vi "Find RetVal Wire_UNUSED.vi"(8 "Error In":errorcluster, 11 "Proto Method VI":refnum<vi>) -> (0 "Error Out":errorcluster, 2 "RetVal Wire":refnum<vi>, 3 "Proto Method VI Dup":refnum<vi>)   [LabVIEW 2013, in "Abstract Param Writer.lvclass"]
uses:
  Abstract Param Writer.lvclass
  <vilib>/Utility/traverseref.llb/TRef TravTarget.ctl
  <vilib>/Utility/traverseref.llb/VI Scripting - Traverse.lvlib
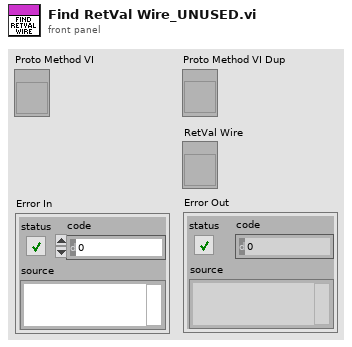
[diagram p1: front panel]
types:
  T1 = typedef "TRef TravTarget.ctl" = enum16{"FP", "BD", "Other"}
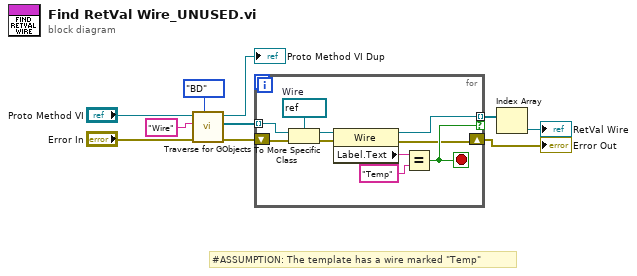
[diagram p0: block diagram]
diagram:
  # "#ASSUMPTION: The template has a wire marked \"Temp\""
  n1 = call <vilib>:"Traverse for GObjects.vi"("Traverse Target"=TRef_TravTarget."BD", "error in (no error)"="Error In", "Class Name"="Wire", "VI Refnum"="Proto Method VI") -> ("error out"=w4:errorcluster, "References"=w6:refnum<vi>[], "dup VI Refnum"=→"Proto Method VI Dup":refnum<vi>)  [unwired: 4 in, 1 out]
  n2 = for {
    tunnel: w6 -> [w20] mode=indexing
    tunnel: [w15] -> w5 mode=indexing if=w14
    shift-right: [w11] -> w1
    shift-left: w4 -> [w12]
    stop <- w14 stop-if-true
    w19 = refnum<vi> refnum  # Wire
    n3 = To More Specific Class(target class=w19, reference=w20, error in=w12) -> (specific class reference=w18:refnum<vi>, error out=w13:errorcluster)
    n4 = property class="Wire"(reference=w18, error in=w13) -> (reference out=w15:refnum<vi>, error out=w11:errorcluster, "Label.Text"=w17:string)
    n5 = Equal?(x=w17, y="Temp") -> (x = y?=w14:bool)
  }
  "Error Out" <- w1
  n6 = Index Array(array=w5) -> (element=→"RetVal Wire":refnum<vi>)  [unwired: 1 in]
